vi "Aquire Image.vi"(8 "error in (no error)":errorcluster, 9 "Cluster":T1={"Gamma::Value"=1.6, "Gain::Value"=50, "Sharpness::Value"=0, "Contrast::Value"=0.5, "Exposure::Value"=0.0078125} {"Exposure::Value" min=0.000244140625 max=0.5; "Contrast::Value" min=0.0 max=1.0; "Sharpness::Value" min=0 max=2 step=1; "Gain::Value" min=0 max=100 step=1; "Gamma::Value" min=0.01 max=10.0}, 10 "Stop":bool, 11 "Edmund Optics in":refnum<class "Edmund Optics.lvclass">) -> (0 "error out":errorcluster, 2 "Image Out":T2(plugin-control), 3 "Edmund Optics out":refnum<class "Edmund Optics.lvclass">)   [LabVIEW 2018, in "Edmund Optics.lvclass"]
uses:
  Edmund Optics.lvclass
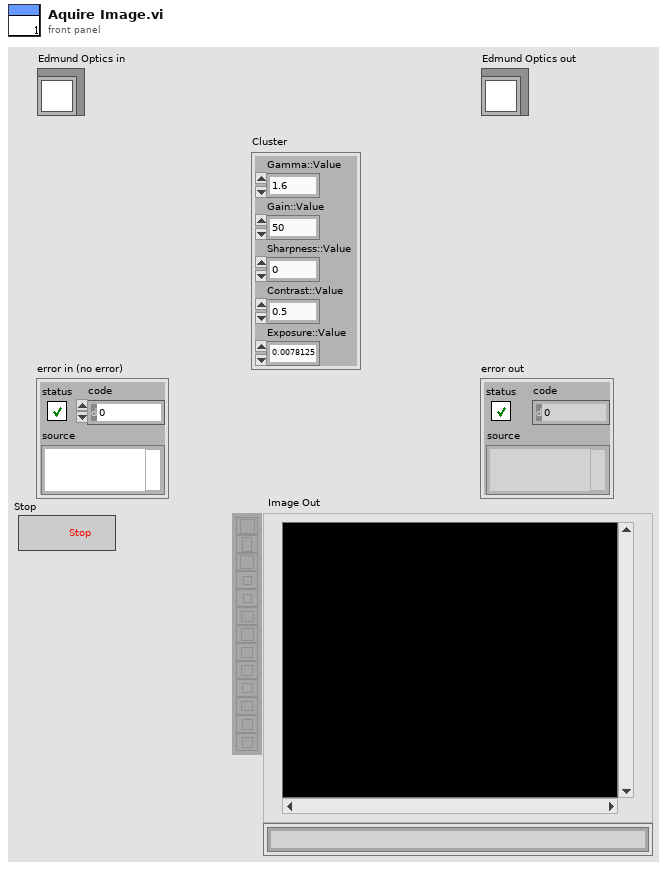
[diagram p1: front panel]
types:
  T1 = cluster{"Gamma::Value":dbl, "Gain::Value":i64, "Sharpness::Value":i64, "Contrast::Value":dbl, "Exposure::Value":dbl}
  T2 = typedef "IMAQ Image.ctl" = refnum<image>
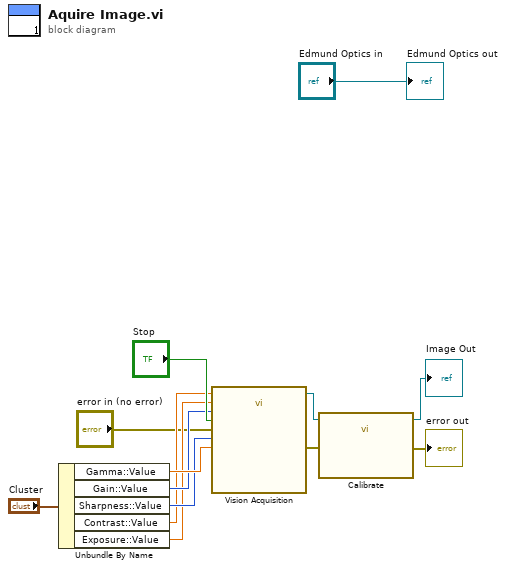
[diagram p0: block diagram]
diagram:
  n1 = Unbundle By Name("Cluster") -> ("Gamma::Value"=w8:dbl, "Gain::Value"=w7:i64, "Sharpness::Value"=w6:i64, "Contrast::Value"=w5:dbl, "Exposure::Value"=w4:dbl)
  n2 = call "Vision Acquisition"("Contrast::Value"=w5, "Exposure::Value"=w4, "Gain::Value"=w7, "Stop (F)"="Stop", "error in"="error in (no error)", "Gamma::Value"=w8, "Sharpness::Value"=w6) -> ("Image Out"=w11:T2, "error out"=w2:errorcluster)  [unwired: 18 in, 1 out]
  n3 = call "Calibrate"("Image In"=w11, "error in"=w2) -> ("Image Out"=→"Image Out":T2, "error out"=→"error out":errorcluster)  [unwired: 24 in]
  "Edmund Optics out" <- "Edmund Optics in"
